vi "Motor Diagnostics.vi"() -> ()   [LabVIEW 2018]
uses:
  <vilib>/Rock Robotics/Network Tables/NT Write Numeric Array.vi
panel:
  out "Front Left to Right":dbl(knob) scale=-50.0..50.0
  out "BRD Current":dbl
  out "BLD Velocity":dbl
  out "BRD Position":dbl
  out "BRD Applied Output":dbl
  out "BRD Voltage":dbl
  out "BRD Temperature":u8
  out "BLD Current":dbl
  out "BLD Velocity":dbl
  out "BLD Position":dbl
  out "BLD Applied Output":dbl
  out "BLD Voltage":dbl
  out "BLD Temperature":u8
  out "FRD Current":dbl
  out "FLD Velocity":dbl
  out "FRD Position":dbl
  out "FRD Applied Output":dbl
  out "FRD Voltage":dbl
  out "FRD Temperature":u8
  out "FLD Current":dbl
  out "FLD Velocity":dbl
  out "FLD Position":dbl
  out "FLD Applied Output":dbl
  out "FLD Voltage":dbl
  out "FLD Temperature":u8
  # "Spark MAX motors"
  # "Front Left Drive"
  # "Front Right Drive"
  # "Black Left Drive"
  # "Black Left Drive"
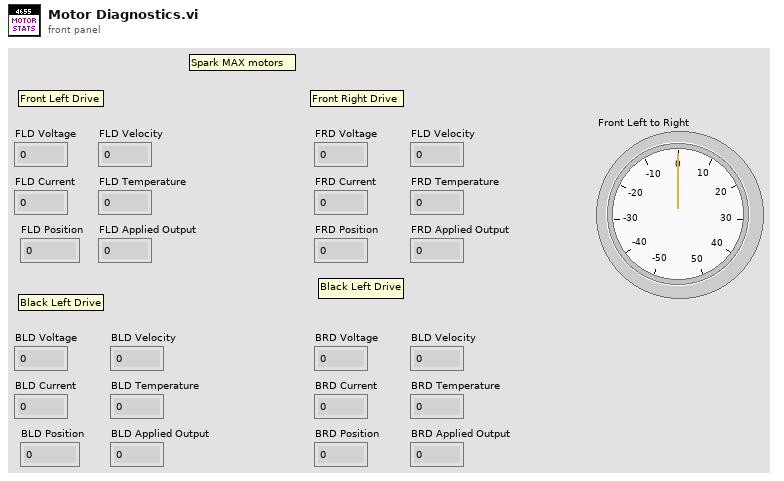
[diagram p1: front panel]
types:
  T1 = typedef "WPI_MotorControlDeviceRef.ctl" = cluster{"DeviceStatus":errorcluster, "Type":T2, "PWM":cluster{"PWM Channel":T3, "DeadBand":T4}, "CAN":cluster{"Device Number":u8, "SetOutput VI Ref":variant, "GetOutput VI Ref":variant, "Enable VI Ref":variant, "Disable VI Ref":variant, "Data":variant}, "Invert":bool, "DIO PWM":cluster{"PWM \"Enable\" Channel":T3, "DIOChannel":T5, "PWM Rate":dbl}}
  T2 = typedef "WPI_MotorControlType.ctl" = enum16{"PWM", "CAN", "DIO PWM"}
  T3 = typedef "FPGA_DIOPWMChannel.ctl" = enum8{"PWM 0", "PWM 1", "PWM 2", "PWM 3", "PWM 4", "PWM 5", "PWM 6", "PWM 7", "PWM 8", "PWM 9", "PWM MXP 0", "PWM MXP 1", "PWM MXP 2", "PWM MXP 3", "PWM MXP 4", "PWM MXP 5", "PWM MXP 6", "PWM MXP 7", "PWM MXP 8", "PWM MXP 9", "Invalid"}
  T4 = typedef "WPI_PWMDeadband.ctl" = cluster{"Name":string, "maxPositivePwm":i32, "minPositivePwm":i32, "centerPwm":i32, "maxNegativePwm":i32, "minNegativePwm":i32, "angularRange":u16}
  T5 = typedef "FPGA_DIOChannel.ctl" = enum8{"DIO 0", "DIO 1", "DIO 2", "DIO 3", "DIO 4", "DIO 5", "DIO 6", "DIO 7", "DIO 8", "DIO 9", "DIO MXP 0", "DIO MXP 1", "DIO MXP 2", "DIO MXP 3", "DIO MXP 4", "DIO MXP 5", "DIO MXP 6", "DIO MXP 7", "DIO MXP 8", "DIO MXP 9", "DIO MXP 10", "DIO MXP 11", "DIO MXP 12", "DIO MXP 13", "DIO MXP 14", "DIO MXP 15", "SPI Port CS1", "SPI Port CS2", "SPI Port CS3", "SPI Port MISO", "SPI Port MOSI", "Invalid"}
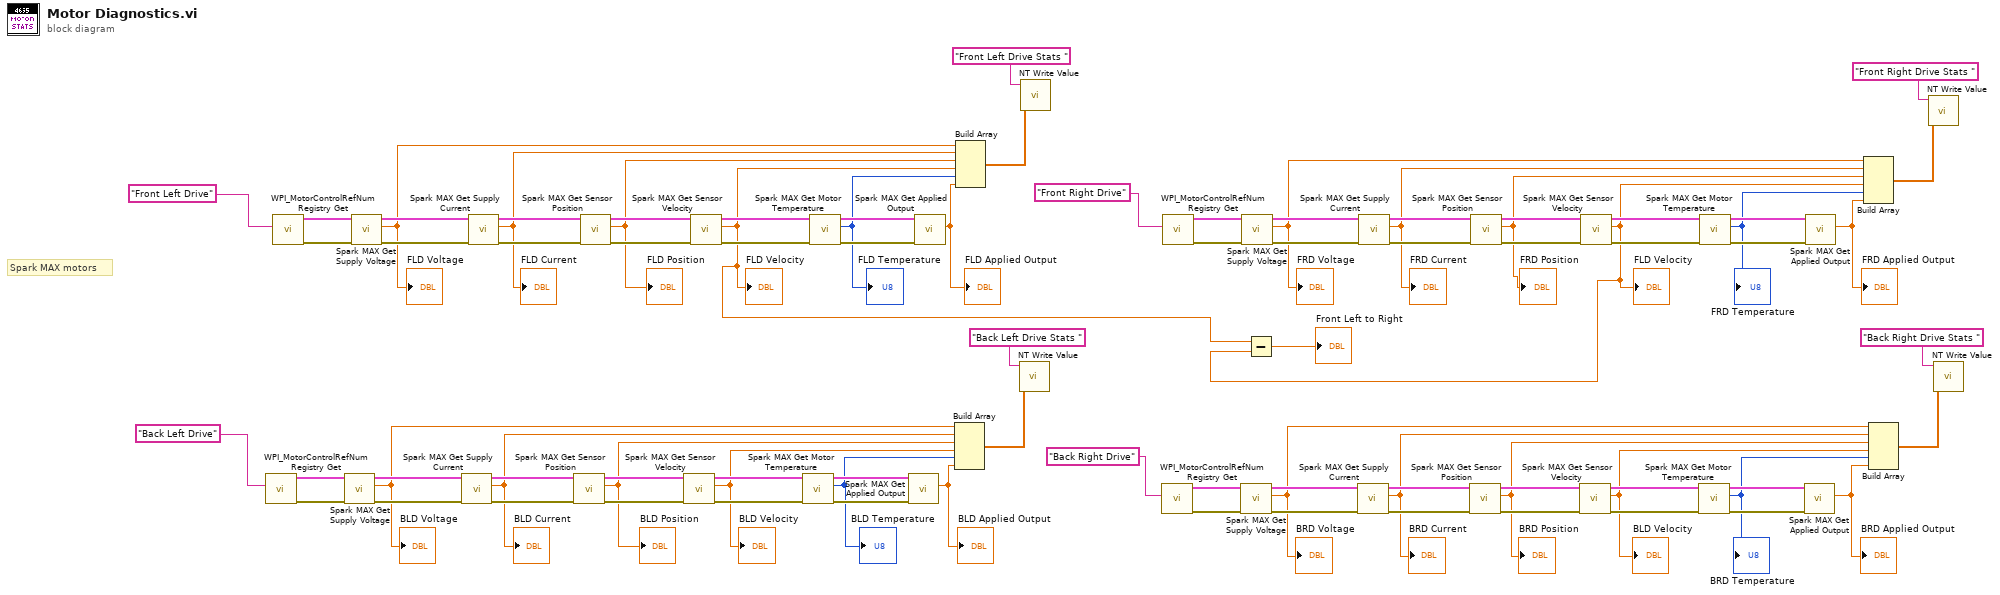
[diagram p0: block diagram]
diagram:
  # "Spark MAX motors"
  n1 = call <vilib>:"WPI_MotorControlRefNum Registry Get.vi"("refnum name"="Back Left Drive") -> ("error out"=w54:errorcluster, "MotorControlDevRef"=w53:T1)  [unwired: 9 in]
  n2 = call <vilib>:"WPI_MotorControlRefNum Registry Get.vi"("refnum name"="Front Left Drive") -> ("error out"=w79:errorcluster, "MotorControlDevRef"=w78:T1)  [unwired: 9 in]
  n3 = call <vilib>:"Spark MAX Get Supply Voltage.vi"("error in (no error)"=w54, "MotorControlDevRef in"=w53) -> ("error out"=w51:errorcluster, "Voltage"=w21:dbl, "MotorControlDevRef out"=w52:T1)  [unwired: 6 in, 1 out]
  "BLD Voltage" <- w21
  n4 = call <vilib>:"Spark MAX Get Supply Voltage.vi"("error in (no error)"=w79, "MotorControlDevRef in"=w78) -> ("error out"=w76:errorcluster, "Voltage"=w36:dbl, "MotorControlDevRef out"=w77:T1)  [unwired: 6 in, 1 out]
  "FLD Voltage" <- w36
  n5 = call <vilib>:"Spark MAX Get Supply Current.vi"("error in (no error)"=w51, "MotorControlDevRef in"=w52) -> ("error out"=w59:errorcluster, "Current"=w20:dbl, "MotorControlDevRef out"=w60:T1)  [unwired: 6 in, 1 out]
  "BLD Current" <- w20
  n6 = call <vilib>:"Spark MAX Get Supply Current.vi"("error in (no error)"=w76, "MotorControlDevRef in"=w77) -> ("error out"=w84:errorcluster, "Current"=w34:dbl, "MotorControlDevRef out"=w85:T1)  [unwired: 6 in, 1 out]
  "FLD Current" <- w34
  n7 = call <vilib>:"Spark MAX Get Sensor Position.vi"("error in (no error)"=w59, "MotorControlDevRef in"=w60) -> ("error out"=w57:errorcluster, "Sensor Position"=w19:dbl, "MotorControlDevRef out"=w58:T1)  [unwired: 6 in, 1 out]
  "BLD Position" <- w19
  n8 = call <vilib>:"Spark MAX Get Sensor Position.vi"("error in (no error)"=w84, "MotorControlDevRef in"=w85) -> ("error out"=w82:errorcluster, "Sensor Position"=w33:dbl, "MotorControlDevRef out"=w83:T1)  [unwired: 6 in, 1 out]
  "FLD Position" <- w33
  n9 = call <vilib>:"Spark MAX Get Sensor Velocity.vi"("error in (no error)"=w57, "MotorControlDevRef in"=w58) -> ("error out"=w49:errorcluster, "Sensor Velocity"=w18:dbl, "MotorControlDevRef out"=w50:T1)  [unwired: 6 in, 1 out]
  "BLD Velocity" <- w18
  n10 = call <vilib>:"Spark MAX Get Sensor Velocity.vi"("error in (no error)"=w82, "MotorControlDevRef in"=w83) -> ("error out"=w74:errorcluster, "Sensor Velocity"=w2:dbl, "MotorControlDevRef out"=w75:T1)  [unwired: 6 in, 1 out]
  "FLD Velocity" <- w2
  n11 = call <vilib>:"Spark MAX Get Motor Temperature.vi"("error in (no error)"=w49, "MotorControlDevRef in"=w50) -> ("error out"=w55:errorcluster, "Motor Temperature"=w17:u8, "MotorControlDevRef out"=w56:T1)  [unwired: 6 in, 1 out]
  "BLD Temperature" <- w17
  n12 = call <vilib>:"Spark MAX Get Motor Temperature.vi"("error in (no error)"=w74, "MotorControlDevRef in"=w75) -> ("error out"=w80:errorcluster, "Motor Temperature"=w32:u8, "MotorControlDevRef out"=w81:T1)  [unwired: 6 in, 1 out]
  "FLD Temperature" <- w32
  n13 = call <vilib>:"Spark MAX Get Applied Output.vi"("error in (no error)"=w55, "MotorControlDevRef in"=w56) -> ("Applied Output"=w16:dbl)  [unwired: 6 in, 3 out]
  "BLD Applied Output" <- w16
  n14 = call <vilib>:"Spark MAX Get Applied Output.vi"("error in (no error)"=w80, "MotorControlDevRef in"=w81) -> ("Applied Output"=w31:dbl)  [unwired: 6 in, 3 out]
  "FLD Applied Output" <- w31
  n15 = Build Array(w21, w20, w19, w18, w17, w16) -> (w22:dbl[])
  n16 = Build Array(w36, w34, w33, w2, w32, w31) -> (w35:dbl[])
  n17 = call-poly <vilib>:"NT Write Value.vi"("Numeric Array"=w22, "Name"="Back Left Drive Stats " ("refnum name")) -> ()  [unwired: 9 in, 1 out]
  n18 = call-poly <vilib>:"NT Write Value.vi"("Numeric Array"=w35, "Name"="Front Left Drive Stats " ("refnum name")) -> ()  [unwired: 9 in, 1 out]
  n19 = call <vilib>:"WPI_MotorControlRefNum Registry Get.vi"("refnum name"="Back Right Drive") -> ("error out"=w42:errorcluster, "MotorControlDevRef"=w41:T1)  [unwired: 9 in]
  n20 = call <vilib>:"WPI_MotorControlRefNum Registry Get.vi"("refnum name"="Front Right Drive") -> ("error out"=w66:errorcluster, "MotorControlDevRef"=w65:T1)  [unwired: 9 in]
  n21 = call <vilib>:"Spark MAX Get Supply Voltage.vi"("error in (no error)"=w42, "MotorControlDevRef in"=w41) -> ("error out"=w39:errorcluster, "Voltage"=w13:dbl, "MotorControlDevRef out"=w40:T1)  [unwired: 6 in, 1 out]
  "BRD Voltage" <- w13
  n22 = call <vilib>:"Spark MAX Get Supply Voltage.vi"("error in (no error)"=w66, "MotorControlDevRef in"=w65) -> ("error out"=w63:errorcluster, "Voltage"=w28:dbl, "MotorControlDevRef out"=w64:T1)  [unwired: 6 in, 1 out]
  "FRD Voltage" <- w28
  n23 = call <vilib>:"Spark MAX Get Supply Current.vi"("error in (no error)"=w39, "MotorControlDevRef in"=w40) -> ("error out"=w47:errorcluster, "Current"=w12:dbl, "MotorControlDevRef out"=w48:T1)  [unwired: 6 in, 1 out]
  "BRD Current" <- w12
  n24 = call <vilib>:"Spark MAX Get Supply Current.vi"("error in (no error)"=w63, "MotorControlDevRef in"=w64) -> ("error out"=w71:errorcluster, "Current"=w27:dbl, "MotorControlDevRef out"=w72:T1)  [unwired: 6 in, 1 out]
  "FRD Current" <- w27
  n25 = call <vilib>:"Spark MAX Get Sensor Position.vi"("error in (no error)"=w47, "MotorControlDevRef in"=w48) -> ("error out"=w45:errorcluster, "Sensor Position"=w11:dbl, "MotorControlDevRef out"=w46:T1)  [unwired: 6 in, 1 out]
  "BRD Position" <- w11
  n26 = call <vilib>:"Spark MAX Get Sensor Position.vi"("error in (no error)"=w71, "MotorControlDevRef in"=w72) -> ("error out"=w69:errorcluster, "Sensor Position"=w26:dbl, "MotorControlDevRef out"=w70:T1)  [unwired: 6 in, 1 out]
  "FRD Position" <- w26
  n27 = call <vilib>:"Spark MAX Get Sensor Velocity.vi"("error in (no error)"=w45, "MotorControlDevRef in"=w46) -> ("error out"=w37:errorcluster, "Sensor Velocity"=w10:dbl, "MotorControlDevRef out"=w38:T1)  [unwired: 6 in, 1 out]
  "BLD Velocity" <- w10
  n28 = call <vilib>:"Spark MAX Get Sensor Velocity.vi"("error in (no error)"=w69, "MotorControlDevRef in"=w70) -> ("error out"=w61:errorcluster, "Sensor Velocity"=w3:dbl, "MotorControlDevRef out"=w62:T1)  [unwired: 6 in, 1 out]
  "FLD Velocity" <- w3
  n29 = Subtract(x=w2, y=w3) -> (x-y=→"Front Left to Right":dbl)
  n30 = call <vilib>:"Spark MAX Get Motor Temperature.vi"("error in (no error)"=w37, "MotorControlDevRef in"=w38) -> ("error out"=w43:errorcluster, "Motor Temperature"=w9:u8, "MotorControlDevRef out"=w44:T1)  [unwired: 6 in, 1 out]
  "BRD Temperature" <- w9
  n31 = call <vilib>:"Spark MAX Get Motor Temperature.vi"("error in (no error)"=w61, "MotorControlDevRef in"=w62) -> ("error out"=w67:errorcluster, "Motor Temperature"=w25:u8, "MotorControlDevRef out"=w68:T1)  [unwired: 6 in, 1 out]
  "FRD Temperature" <- w25
  n32 = call <vilib>:"Spark MAX Get Applied Output.vi"("error in (no error)"=w43, "MotorControlDevRef in"=w44) -> ("Applied Output"=w8:dbl)  [unwired: 6 in, 3 out]
  "BRD Applied Output" <- w8
  n33 = call <vilib>:"Spark MAX Get Applied Output.vi"("error in (no error)"=w67, "MotorControlDevRef in"=w68) -> ("Applied Output"=w24:dbl)  [unwired: 6 in, 3 out]
  "FRD Applied Output" <- w24
  n34 = Build Array(w28, w27, w26, w3, w25, w24) -> (w29:dbl[])
  n35 = Build Array(w13, w12, w11, w10, w9, w8) -> (w14:dbl[])
  n36 = call-poly <vilib>:"NT Write Value.vi"("Numeric Array"=w29, "Name"="Front Right Drive Stats " ("refnum name")) -> ()  [unwired: 9 in, 1 out]
  n37 = call-poly <vilib>:"NT Write Value.vi"("Numeric Array"=w14, "Name"="Back Right Drive Stats " ("refnum name")) -> ()  [unwired: 9 in, 1 out]
